vi "生成word报表.vi"(7 "类型":string, 8 "部位":string, 9 "测试人":string, 10 "产品序号":string, 11 "Array输入":refnum<vi>) -> (3 "报告生成路径":path)   [LabVIEW 2018]
uses:
  <vilib>/Utility/NIReport.llb/Report Type.ctl
  <vilib>/Utility/NIReport.llb/Append Report Text (str wrap).vi
  <vilib>/addons/_office/word.llb/Word Edit Cell ([dbl]).vi
  <vilib>/Utility/NIReport.llb/NI_report.lvclass
  <vilib>/addons/_office/NI_ReportGenerationToolkit.lvlib
  <vilib>/Utility/NIReport.llb/Word/NI_Word.lvclass
  <vilib>/Utility/NIReport.llb/NI_ReportGenerationCore.lvlib
panel:
  out "缺陷个数":i32
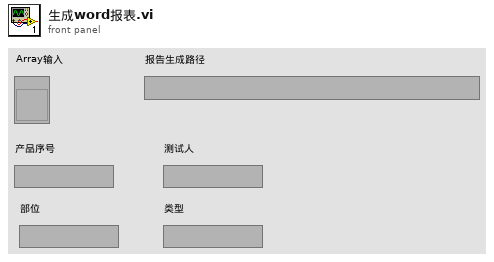
[diagram p1: front panel]
types:
  T1 = cluster{"position (Excel)":cluster{"row":i32, "column":i32}, "name (Excel)":string, "bookmark (Word)":string}
  T2 = typedef "NI_ReportGenerationCore.lvlib/Report Type.ctl" = enum16{"HTML", "Word", "Excel"}
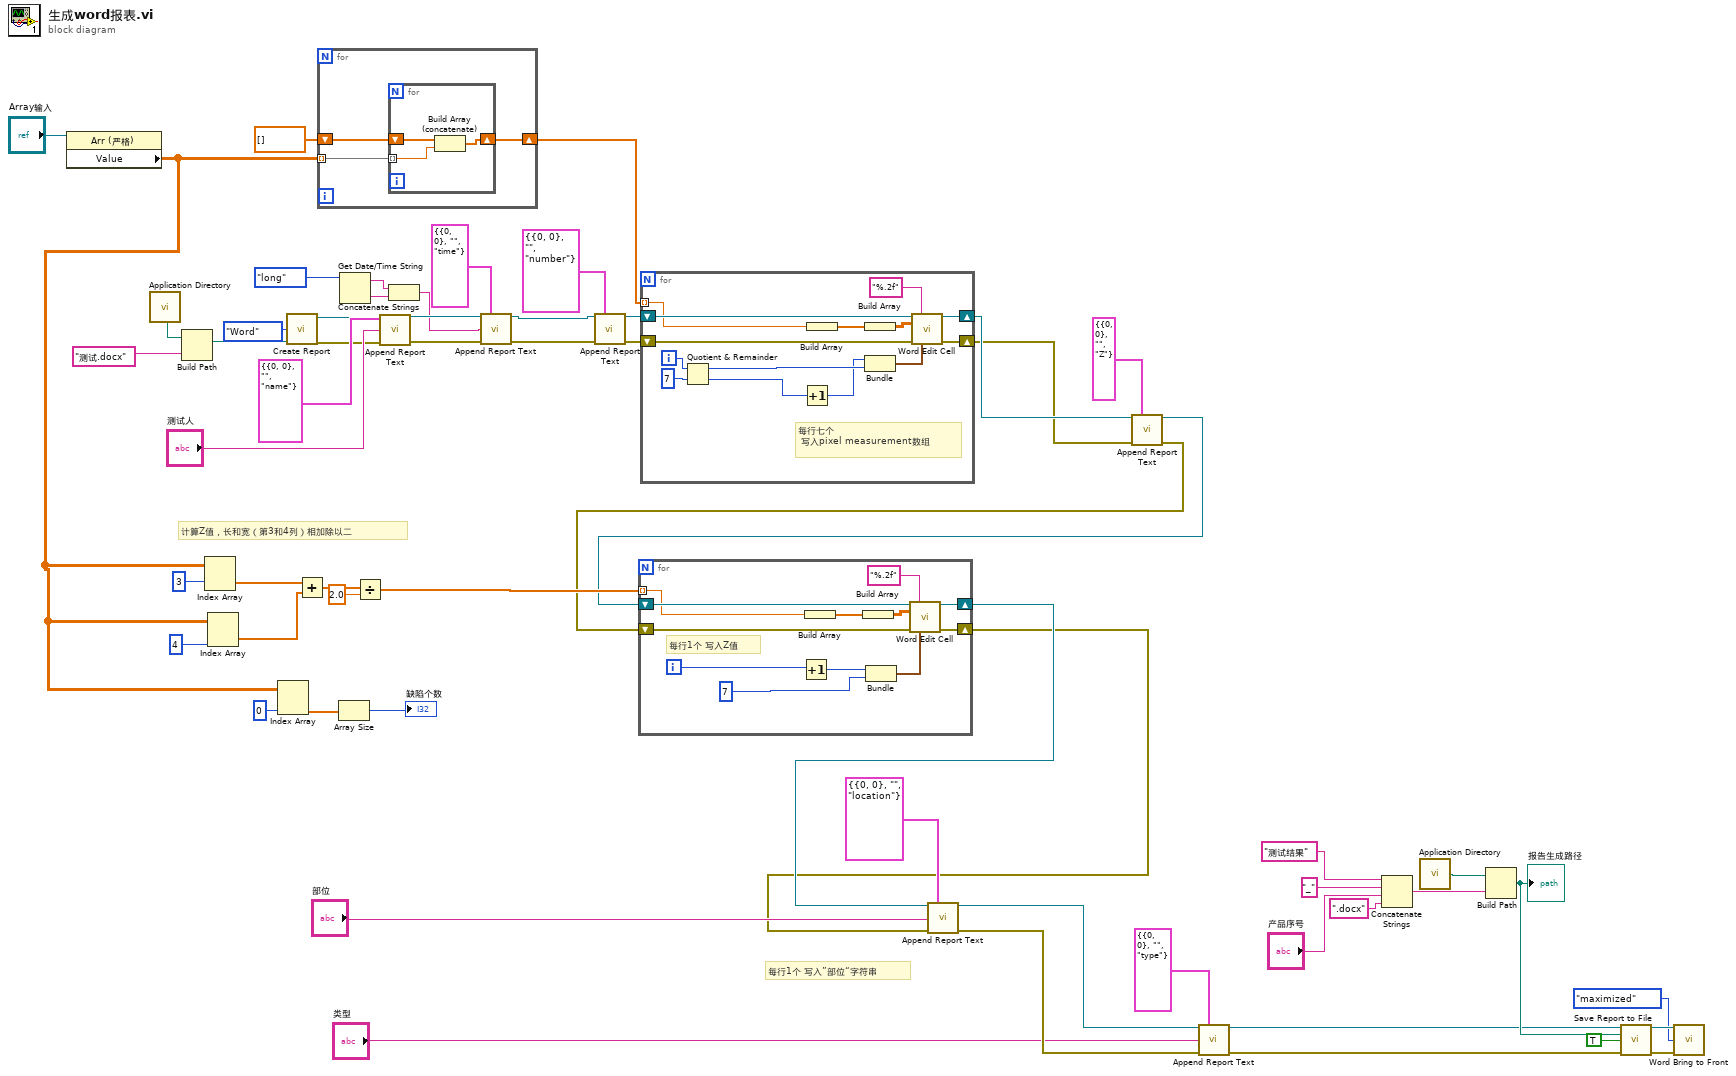
[diagram p0: block diagram]
diagram:
  # "每行1个 写入”部位“字符串"
  # "计算Z值，长和宽（第3和4列）相加除以二"
  n1 = property class="Arr (严格)"(reference="Array输入") -> ("Value"=w12:dbl[][])  [unwired: 1 in, 2 out]
  n2 = call <vilib>:"Application Directory.vi"() -> ("Application Directory"=w29:path)
  n3 = Build Path(base path=w29, name or relative path="测试.docx") -> (appended path=w32:path)
  n4 = Index Array(array=w12, index (col)=3 ("索引")) -> (element=w27:dbl[])  [unwired: 1 in]
  n5 = Index Array(array=w12, index (col)=4 ("索引")) -> (element=w26:dbl[])  [unwired: 1 in]
  n6 = Index Array(array=w12, index (col)=0 ("禁用的索引 (列)")) -> (element=w14:dbl[])  [unwired: 1 in]
  n7 = call <vilib>:"Create Report.vi"("report type"=Report_Type."Word" ("Report Type"), "template (empty)"=w32) -> ("report out"=w55:refnum<class "NI_report.lvclass">, "error out"=w58:errorcluster)  [unwired: 12 in]
  n8 = Add(x=w27, y=w26) -> (x+y=w25:dbl[])
  n9 = for {
    tunnel: w12 -> [w63] mode=indexing
    shift-right: [w61] -> w53
    shift-left: dbl[] [] ("元素") -> [w62]
    n10 = for {
      tunnel: w63 -> [w66] mode=indexing
      shift-right: [w64] -> w61
      shift-left: w62 -> [w65]
      n11 = Build Array (concatenate)(w65, w66) -> (w64:dbl[])
    }
  }
  n12 = Array Size(array=w14) -> (size(s)=→"缺陷个数":i32)
  n13 = Get Date/Time String(date format (0)=enum16{"short", "long", "abbreviated"}."long" ("日期格式(0)")) -> (date string=w33:string, time string=w35:string)  [unwired: 2 in]
  n14 = Divide(x=w25, y=2.0) -> (x/y=w20:dbl[])
  n15 = call-poly <vilib>:"Append Report Text.vi"("report in"=w55, "MS Office parameters"=T1 {"position (Excel)"={"row"=0, "column"=0}, "name (Excel)"="", "bookmark (Word)"="name"}, "text"="测试人", "error in (no error)"=w58) -> ("report out"=w56:refnum<class "NI_report.lvclass">, "error out"=w57:errorcluster)  [unwired: 8 in, 2 out]
  n16 = Concatenate Strings(w33, w35) -> (w34:string)
  n17 = call-poly <vilib>:"Append Report Text.vi"("report in"=w56, "MS Office parameters"=T1 {"position (Excel)"={"row"=0, "column"=0}, "name (Excel)"="", "bookmark (Word)"="time"}, "text"=w34, "error in (no error)"=w57) -> ("report out"=w48:refnum<class "NI_report.lvclass">, "error out"=w49:errorcluster)  [unwired: 8 in, 2 out]
  n18 = call-poly <vilib>:"Append Report Text.vi"("report in"=w48, "MS Office parameters"=T1 {"position (Excel)"={"row"=0, "column"=0}, "name (Excel)"="", "bookmark (Word)"="number"}, "error in (no error)"=w49) -> ("report out"=w50:refnum<class "NI_report.lvclass">, "error out"=w51:errorcluster)  [unwired: 9 in, 2 out]
  n19 = for {
    shift-right: [w80] -> w18
    shift-left: w50 -> [w75]
    shift-right: [w79] -> w17
    shift-left: w51 -> [w74]
    tunnel: w53 -> [w68] mode=indexing
    i -> [w76]
    # "每行七个\n 写入pixel measurement数组"
    n20 = Quotient & Remainder(x=w76, y=7) -> (x-y*floor(x/y)=w73:i32, floor(x/y)=w72:i32)
    n21 = Increment(x=w72) -> (x+1=w71:i32)
    n22 = Build Array(w68) -> (w70:dbl[])
    n23 = Build Array(w70) -> (w69:dbl[][])
    n24 = Bundle(w71, w73) -> (w78:cluster{i32, i32})  [unwired: 1 in]
    n25 = call-poly <vilib>:"Word Edit Cell.vi"("report in"=w75, "format string (%.3f)"="%.2f", "value"=w69, "error in (no error)"=w74, "start (0, 0)"=w78) -> ("report out"=w80:refnum<class "NI_report.lvclass">, "error out"=w79:errorcluster)  [unwired: 9 in]
  }
  n26 = call-poly <vilib>:"Append Report Text.vi"("report in"=w18, "MS Office parameters"=T1 {"position (Excel)"={"row"=0, "column"=0}, "name (Excel)"="", "bookmark (Word)"="Z"}, "error in (no error)"=w17) -> ("report out"=w16:refnum<class "NI_report.lvclass">, "error out"=w15:errorcluster)  [unwired: 9 in, 2 out]
  n27 = for {
    shift-right: [w92] -> w5
    shift-left: w16 -> [w89]
    shift-right: [w91] -> w4
    shift-left: w15 -> [w88]
    tunnel: w20 -> [w84] mode=indexing
    i -> [w82]
    # "每行1个 写入Z值"
    n28 = Increment(x=w82) -> (x+1=w87:i32)
    n29 = Build Array(w84) -> (w86:dbl[])
    n30 = Build Array(w86) -> (w85:dbl[][])
    n31 = Bundle(w87, "y"=7) -> (w90:cluster{i32, "y":i32})  [unwired: 1 in]
    n32 = call-poly <vilib>:"Word Edit Cell.vi"("report in"=w89, "format string (%.3f)"="%.2f", "value"=w85, "error in (no error)"=w88, "start (0, 0)"=w90) -> ("report out"=w92:refnum<class "NI_report.lvclass">, "error out"=w91:errorcluster)  [unwired: 9 in]
  }
  n33 = call-poly <vilib>:"Append Report Text.vi"("report in"=w5, "MS Office parameters"=T1 {"position (Excel)"={"row"=0, "column"=0}, "name (Excel)"="", "bookmark (Word)"="location"}, "text"="部位", "error in (no error)"=w4) -> ("report out"=w7:refnum<class "NI_report.lvclass">, "error out"=w8:errorcluster)  [unwired: 8 in, 2 out]
  n34 = call-poly <vilib>:"Append Report Text.vi"("report in"=w7, "MS Office parameters"=T1 {"position (Excel)"={"row"=0, "column"=0}, "name (Excel)"="", "bookmark (Word)"="type"}, "text"="类型", "error in (no error)"=w8) -> ("report out"=w2:refnum<class "NI_report.lvclass">, "error out"=w1:errorcluster)  [unwired: 8 in, 2 out]
  n35 = Concatenate Strings("测试结果" ("字符串"), "_" ("名称或相对路径"), "产品序号", ".docx" ("名称或相对路径")) -> (w40:string)
  n36 = call <vilib>:"Application Directory.vi"() -> ("Application Directory"=w39:path)
  n37 = Build Path(base path=w39, name or relative path=w40) -> (appended path=w21:path)
  "报告生成路径" <- w21
  n38 = call-dynamic "Save Report to File.vi"("report in"=w2, "report file path"=w21, "prompt to replace? (F)"=TRUE, "error in (no error)"=w1) -> ("report out"=w45:refnum<class "NI_report.lvclass">, "error out"=w46:errorcluster)  [unwired: 10 in]
  n39 = call <vilib>:"Word Bring to Front.vi"("report in"=w45, "window state (maximized)"=enum16{"maximized", "minimized", "normal"}."maximized", "error in (no error)"=w46) -> ()  [unwired: 11 in, 2 out]
